vi "Main.vi"   [LabVIEW 2020, in "StashRoyale.lvclass"]
uses:
  StashRoyale.lvclass
  7f731695-109d-409f-ac0d-93f72082f8bc.vi
  99389695-3719-4ef4-b472-a74a062ab17b.vi
  78007402-5af3-4aa4-adf5-8423a01fd2ea.vi
  96293f5f-0260-40d0-a2c2-fd21f77f43e5.vi
  support/Popup Loading Toolkit.lvlibp/Handler/Popup Loading Handler.lvclass
types:
  T1 = typedef "StashRoyale.lvclass/InitParameters.ctl" = cluster{"PlayerTag":string, "DBPath":path}
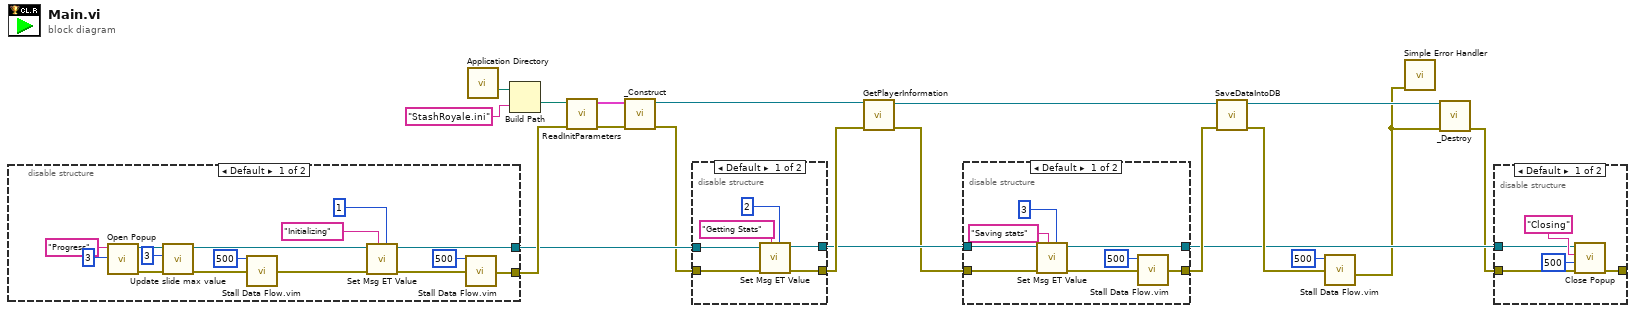
[diagram p0: block diagram]
diagram:
  n1 = disable-structure shown="Default" {
    disable-tunnel: [w22 w36] -> w15
    disable-tunnel: [w21 _] -> w14
    frame condition #0 (active) {
      n2 = call "Open Popup.vi"("Nb Steps"=u32 3, "Title"="Progress") -> ("error out"=w31:errorcluster, "Popup Loading Handler out"=w30:refnum<class "Popup Loading Handler.lvclass">)  [unwired: 8 in]
      n3 = call "Update slide max value.vi"("error in (no error)"=w31, "Slide Max"=u32 3, "Popup Loading Handler in"=w30) -> ("error out"=w28:errorcluster, "Popup Loading Handler out"=w26:refnum<class "Popup Loading Handler.lvclass">)  [unwired: 7 in]
      n4 = call "Stall Data Flow.vim"("value in"=w28, "milliseconds to wait"=u32 500) -> ("value out"=w25:errorcluster)  [unwired: 1 out]
      n5 = call "Set Msg ET Value.vi"("New Value"=u32 1, "New Message"="Initializing", "error in (no error)"=w25, "Popup Loading Handler in"=w26) -> ("error out"=w23:errorcluster, "Popup Loading Handler out"=w21:refnum<class "Popup Loading Handler.lvclass">)  [unwired: 6 in]
      n6 = call "Stall Data Flow.vim"("value in"=w23, "milliseconds to wait"=u32 500) -> ("value out"=w22:errorcluster)  [unwired: 1 out]
    }
    frame condition #1 {
    }
  }
  n7 = call <vilib>:"Application Directory.vi"() -> ("Application Directory"=w17:path)
  n8 = Build Path(base path=w17, name or relative path="StashRoyale.ini" ("Title")) -> (appended path=w18:path)
  n9 = call "ReadInitParameters.vi"("error in (no error)"=w15, "INI Filepath"=w18) -> ("error out"=w16:errorcluster, "Init Parameters"=w19:T1)  [unwired: 8 in]
  n10 = call "_Construct.vi"("error in (no error)"=w16, "Init Parameters"=w19) -> ("error out"=w13:errorcluster, "ClashRoyale out"=w11:refnum<class "StashRoyale.lvclass">)  [unwired: 8 in]
  n11 = disable-structure shown="Default" {
    disable-tunnel: w14 -> [w40 w43]
    disable-tunnel: w13 -> [w39 w44]
    disable-tunnel: [w38 w44] -> w12
    disable-tunnel: [w37 w43] -> w10
    frame condition #0 (active) {
      n12 = call "Set Msg ET Value.vi"("New Value"=u32 2, "New Message"="Getting Stats", "error in (no error)"=w39, "Popup Loading Handler in"=w40) -> ("error out"=w38:errorcluster, "Popup Loading Handler out"=w37:refnum<class "Popup Loading Handler.lvclass">)  [unwired: 6 in]
    }
    frame condition #1 {
    }
  }
  n13 = call "GetPlayerInformation.vi"("error in (no error)"=w12, "ClashRoyale in"=w11) -> ("error out"=w9:errorcluster, "ClashRoyale out"=w8:refnum<class "StashRoyale.lvclass">)  [unwired: 8 in]
  n14 = disable-structure shown="Default" {
    disable-tunnel: w10 -> [w50 w53]
    disable-tunnel: w9 -> [w49 w54]
    disable-tunnel: [w46 w54] -> w7
    disable-tunnel: [w45 w53] -> w3
    frame condition #0 (active) {
      n15 = call "Set Msg ET Value.vi"("New Value"=u32 3, "New Message"="Saving stats", "error in (no error)"=w49, "Popup Loading Handler in"=w50) -> ("error out"=w47:errorcluster, "Popup Loading Handler out"=w45:refnum<class "Popup Loading Handler.lvclass">)  [unwired: 6 in]
      n16 = call "Stall Data Flow.vim"("value in"=w47, "milliseconds to wait"=u32 500) -> ("value out"=w46:errorcluster)  [unwired: 1 out]
    }
    frame condition #1 {
    }
  }
  n17 = call "SaveDataIntoDB.vi"("error in (no error)"=w7, "ClashRoyale in"=w8) -> ("error out"=w5:errorcluster, "ClashRoyale out"=w4:refnum<class "StashRoyale.lvclass">)  [unwired: 8 in]
  n18 = call "Stall Data Flow.vim"("value in"=w5, "milliseconds to wait"=u32 500) -> ("value out"=w2:errorcluster)  [unwired: 1 out]
  n19 = call <vilib>:"Simple Error Handler.vi"("error in (no error)"=w2) -> ()  [unwired: 4 in, 5 out]
  n20 = call "_Destroy.vi"("error in (no error)"=w2, "ClashRoyale in"=w4) -> ("error out"=w1:errorcluster)  [unwired: 9 in]
  n21 = disable-structure shown="Default" {
    disable-tunnel: w3 -> [w57 _]
    disable-tunnel: w1 -> [w56 w60]
    disable-tunnel: [w55 w60] -> _
    frame condition #0 (active) {
      n22 = call "Close Popup.vi"("error in (no error)"=w56, "Wait (200 ms)"=u32 500, "Last Message"="Closing", "Popup Loading Handler in"=w57) -> ("error out"=w55:errorcluster)  [unwired: 7 in]
    }
    frame condition #1 {
    }
  }
